vi "FRCts20_Backend_Team_GET.vi"(6 "Message Attributes":T4, 8 "error in (no error)":errorcluster, 10 "Data":string, 11 "Engine_Refnums":T1) -> (0 "error out":errorcluster)   [LabVIEW 2014, in "FRCts20_Backend_Engine.lvlib"]
doc: "Gets all information and requests under a selected team. Called by the Team API, expects a team index"
uses:
  FRCts20_Backend_Engine.lvlib
  Dependencies/Keyed Array/KeyedArray.ctl
  FRCts20_Backend_EngineRefnums.ctl
  INI_Accessor/FRCts20_Backend_INI Controller.lvclass
  Dependencies/AMC/_SubVIs/TypeDefs/Message Queue.ctl
  Dependencies/AMC/_SubVIs/TypeDefs/Message.ctl
  <vilib>/addons/database/Connection.llb/Conn ObjectReference.ctl
  FRCts20_Backend_API/Team.ctl
  FRCts20_Backend_API/ApiReturn.ctl
  FRCts20_Backend_API/TeamRoot.ctl
  FRCts20_Backend_API/FRCts20_Backend_API_SW.ctl
  FRCts20_Backend_API/TeamExtended.ctl
  FRCts20_Backend_API/EventRoot.ctl
  FRCts20_Backend_FGVOperation.ctl
  FRCts20_Backend_API/FRCts20_Backend_API.lvlib
  Dependencies/Keyed Array/Tools_KeyedArray.lvlib
  Dependencies/AMC/AMC.lvlib
  <vilib>/addons/database/NI_Database_API.lvlib
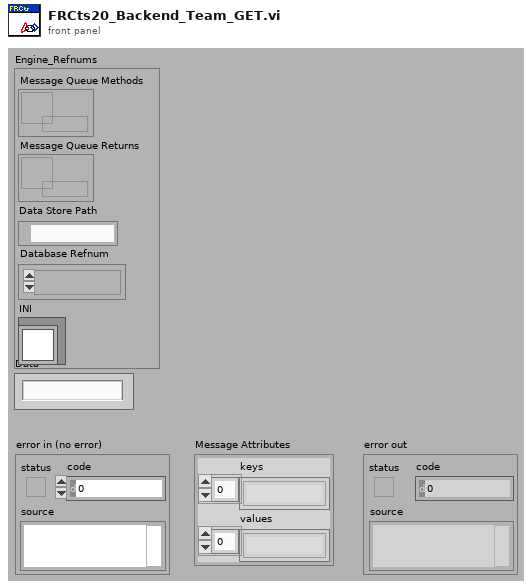
[diagram p1: front panel]
types:
  T1 = typedef "FRCts20_Backend_Engine.lvlib/FRCts20_Backend_EngineRefnums.ctl" = cluster{"Message Queue Methods":T2, "Message Queue Returns":T2, "Data Store Path":path, "Database Refnum":T3, "INI":refnum<class "FRCts20_Backend_INI Controller.lvclass">}
  T2 = typedef "AMC.lvlib/Message Queue.ctl" = refnum<queue>
  T3 = typedef "NI_Database_API.lvlib/Conn ObjectReference.ctl" = refnum<k1>
  T4 = typedef "Tools_KeyedArray.lvlib/KeyedArray.ctl" = cluster{"keys":string[], "values":string[]}
  T5 = typedef "FRCts20_Backend_Engine.lvlib/FRCts20_Backend_FGVOperation.ctl" = enum16{"Initialize", "EnqueueMessage", "EnqueueDataReturn", "FlushMessage", "FlushDataReturn"}
  T6 = typedef "FRCts20_Backend_Engine.lvlib/FRCts20_Backend_API.lvlib/Team.ctl" = cluster{"APIReturn":T7, "TeamRoot":T8, "TeamExtendedData":T10, "Events":T11[]}
  T7 = typedef "FRCts20_Backend_Engine.lvlib/FRCts20_Backend_API.lvlib/ApiReturn.ctl" = string
  T8 = typedef "FRCts20_Backend_Engine.lvlib/FRCts20_Backend_API.lvlib/TeamRoot.ctl" = cluster{"TeamIndex":i32, "TeamNumber":u32, "SoftwareType":T9}
  T9 = typedef "FRCts20_Backend_Engine.lvlib/FRCts20_Backend_API.lvlib/FRCts20_Backend_API_SW.ctl" = string
  T10 = typedef "FRCts20_Backend_Engine.lvlib/FRCts20_Backend_API.lvlib/TeamExtended.ctl" = cluster{"TeamName":string, "ShortTeamName":string, "NickName":string, "RobotName":string, "City":string, "State":string, "Country":string, "RookieYear":u32, "CAN":bool, "Vision":bool, "Kinect":bool, "Avatar":string, "Team ID":u32, "Tags":string}
  T11 = typedef "FRCts20_Backend_Engine.lvlib/FRCts20_Backend_API.lvlib/EventRoot.ctl" = cluster{"EventIndex":i32, "EventName":string, "IsLive":bool, "OpenIssues":i32}
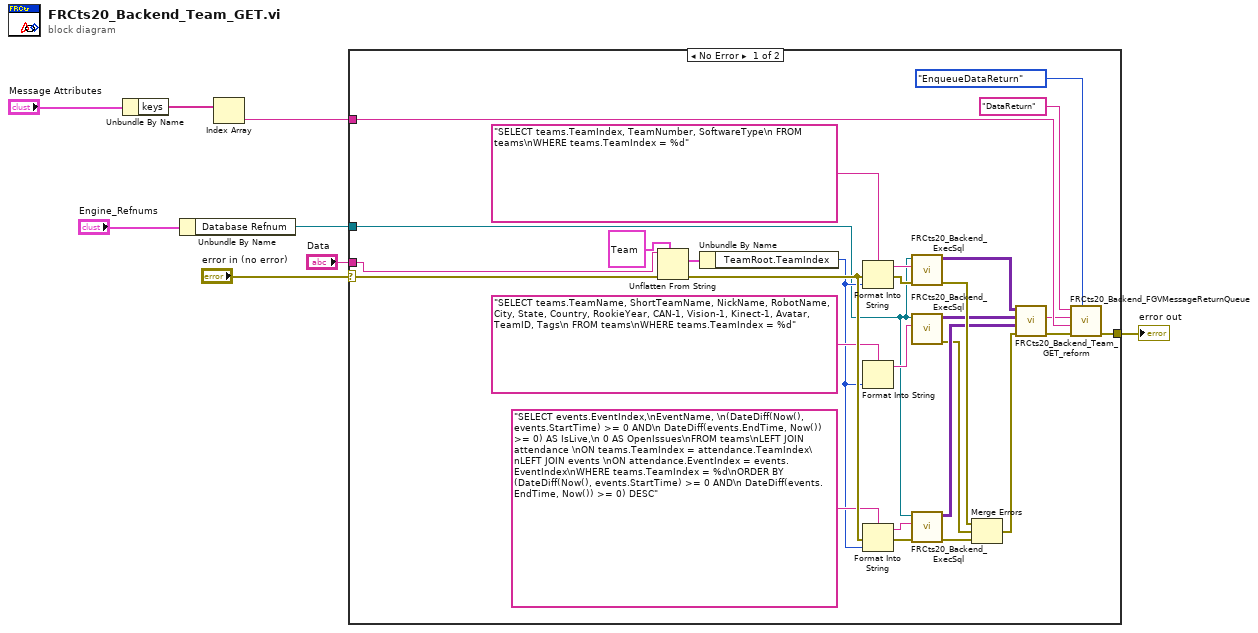
[diagram p0: block diagram]
diagram:
  n1 = Unbundle By Name("Message Attributes") -> ("keys"=w4:string[])
  n2 = Unbundle By Name("Engine_Refnums") -> ("Database Refnum"=w1:T3)
  n3 = Index Array(array=w4) -> (element=w3:string)  [unwired: 1 in]
  n4 = case shown="No Error" "error in (no error)" {
    selector: "error in (no error)" -> [w33 w37]
    tunnel: [w36 w37] -> w7
    tunnel: w1 -> [w13 _]
    tunnel: "Data" -> [w34 _]
    tunnel: w3 -> [w35 _]
    frame No Error {
      n5 = Unflatten From String(type=T6 {"APIReturn"="", "TeamRoot"={"TeamIndex"=0, "TeamNumber"=0, "SoftwareType"=""}, "TeamExtendedData"={"TeamName"="", "ShortTeamName"="", "NickName"="", "RobotName"="", "City"="", "State"="", "Country"="", "RookieYear"=0, "CAN"=FALSE, "Vision"=FALSE, "Kinect"=FALSE, "Avatar"="", "Team ID"=0, "Tags"=""}, "Events"=[]} ("TeamRoot"), binary string=w34, error in (no error)=w33) -> (value=w17:T6, error out=w20:errorcluster)  [unwired: 2 in, 1 out]
      n6 = Unbundle By Name(w17) -> ("TeamRoot.TeamIndex"=w15:i32)
      n7 = Format Into String(format string="SELECT teams.TeamIndex, TeamNumber, SoftwareType\n FROM teams\nWHERE teams.TeamIndex = %d", error in=w20, w15) -> (resulting string=w22:string, error out=w26:errorcluster)  [unwired: 1 in]
      n8 = Format Into String(format string="SELECT teams.TeamName, ShortTeamName, NickName, RobotName, City, State, Country, RookieYear, CAN-1, Vision-1, Kinect-1, Avatar, TeamID, Tags\n FROM teams\nWHERE teams.TeamIndex = %d", w15) -> (resulting string=w14:string)  [unwired: 2 in, 1 out]
      n9 = Format Into String(format string="SELECT events.EventIndex,\nEventName, \n(DateDiff(Now(), events.StartTime) >= 0 AND\n DateDiff(events.EndTime, Now()) >= 0) AS IsLive,\n 0 AS OpenIssues\nFROM teams\nLEFT JOIN attendance \nON teams.TeamIndex = attendance.TeamIndex\nLEFT JOIN events \nON attendance.EventIndex = events.EventIndex\nWHERE teams.TeamIndex = %d\nORDER BY (DateDiff(Now(), events.StartTime) >= 0 AND\n DateDiff(events.EndTime, Now()) >= 0) DESC", error in=w20, w15) -> (resulting string=w18:string, error out=w21:errorcluster)  [unwired: 1 in]
      n10 = call "FRCts20_Backend_ExecSql.vi"("error in (no error)"=w26, "format string"=w22, "Refnum in"=w13) -> ("error out"=w23:errorcluster, "recordset data"=w25:variant[][])  [unwired: 6 in, 1 out]
      n11 = call "FRCts20_Backend_ExecSql.vi"("format string"=w14, "Refnum in"=w13) -> ("error out"=w9:errorcluster, "recordset data"=w10:variant[][])  [unwired: 7 in, 1 out]
      n12 = call "FRCts20_Backend_ExecSql.vi"("error in (no error)"=w21, "format string"=w18, "Refnum in"=w13) -> ("error out"=w12:errorcluster, "recordset data"=w11:variant[][])  [unwired: 6 in, 1 out]
      n13 = Merge Errors(w23, w9, w12) -> (w24:errorcluster)
      n14 = call "FRCts20_Backend_Team_GET_reform.vi"("error in (no error)"=w24, "eventdata"=w11, "teamData"=w10, "teamRootdata"=w25) -> ("error out"=w31:errorcluster, "data string"=w28:string)  [unwired: 6 in]
      n15 = call "FRCts20_Backend_FGVMessageReturnQueue.vi"("Operation"=FRCts20_Backend_FGVOperation."EnqueueDataReturn", "error in (no error)"=w31, "Key"=w35, "Message Value"=w28, "Message Name"="DataReturn") -> ("error out"=w36:errorcluster)  [unwired: 5 in, 1 out]
    }
    frame Error {
    }
  }
  "error out" <- w7
